vi "Control - Intake Air Desired MAF.vi"(8 "Control Inputs":T1={"Engine Speed [RPM]"=0.0, "Engine Status"=enum."STALLED", "Load Control \nMode"=enum."High-Idle Governor", "dt(s)"=0.0, "Number of Cylinders"=0, "Engine Displacement [cc]"=0.0, "StoichAFR"=0.0, "Q.LHV Fuel [kJ/kg]"=0.0, "BattV PSU [V]"=0.0, "12V PSU [V]"=0.0, "5V PSU [V]"=0.0, "Pedal Position [%]"=0.0, "Oil Pressure [kPa]"=0.0, "Oil Temp [C]"=0.0, "Oil Level [%]"=0.0, "Engine Coolant Temp (ECT) [C]"=0.0, "Engine Coolant Pressure [kPa]"=0.0, "Rail Pressure [bar]"=0.0, "Fuel Pressure [kPa]"=0.0, "Fuel Temp [C]"=0.0, "Vacuum Pressure [kPa]"=0.0, "Throttle Position [%]"=0.0, "Cam1 Advance [CAD]"=0.0, "Cam2 Advance [CAD]"=0.0, "CA50 Control Output [CAD]"=[], "CA50 Control Output Valid"=[], "Intake Air Temp (IAT) [C]"=0.0, "Barometric Air Pressure [kPa]"=0.0, "Intake Air Rel. Humidity [%]"=0.0, "Mass Air Flow (MAF) [kg/hr]"=0.0, "Turbo Inlet Air Pressure [kPa]"=0.0, "Turbo Inlet Air Temp [C]"=0.0, "Turbo Outlet Air Pressure [kPa]"=0.0, "Turbo Outlet Air Temp [C]"=0.0, "CAC Outlet Pressure [kPa]"=0.0, "CAC Outlet Temp [C]"=0.0, "Intake Manifold Pressure (MAP) [kPa]"=0.0, "Intake Manifold Temp (MAT) [C]"=0.0, "Exhaust Manifold Pressure [kPa]"=0.0, "Exhaust Manifold Temp [C]"=0.0, "HighP EGR Cooler Outlet Pressure [kPa]"=0.0, "HighP EGR Cooler Outlet Temp [C]"=0.0, "HighP EGR Differential Pressure [kPa]"=0.0, "HighP EGR Valve Position [%]"=0.0, "Turbo Outlet Exhaust Pressure [kPa]"=0.0, "Turbo Outlet Exhaust Temp [C]"=0.0, "VGT Position 1 [%]"=0.0, "VGT Position 2 [%]"=0.0, "Turbo Speed 1 [RPM]"=0.0, "Turbo Speed 2 [RPM]"=0.0, "LowP EGR Differential Pressure [kPa]"=0.0, "LowP EGR Valve Position [%]"=0.0, "UEGO1Lambda"=0.0, "UEGO1_Hot"=FALSE, "UEGO2Lambda"=0.0, "UEGO2_Hot"=FALSE} {"CA50 Control Output [CAD]" format="%.2f"; "VGT Position 1 [%]" format="%.2f"; "Turbo Speed 2 [RPM]" format="%.2f"; "LowP EGR Valve Position [%]" format="%.2f"; "Turbo Inlet Air Temp [C]" format="%#_6f"; "Turbo Outlet Air Temp [C]" format="%#_6f"; "UEGO2Lambda" format="%.2f"; "Turbo Speed 1 [RPM]" format="%.2f"; "UEGO1Lambda" format="%.2f"}, 9 "Volumetric Efficiency [%]":sgl, 11 "MEP Desired [bar]":sgl) -> (0 "Intake MAP Desired [kPa]":sgl, 1 "Air Mass Desired [mg/cyc]":sgl)   [LabVIEW 2015, in "ECS-RT.lvlib"]
uses:
  ECS-RT.lvlib
  Typedefs/Control Inputs/Control Inputs.ctl
  Typedefs/EPT/Engine Status.ctl
  Typedefs/MISC/Load Control Mode.ctl
  ECS-Shared.lvlib
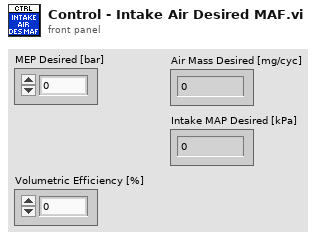
[diagram p1: front panel]
types:
  T1 = typedef "ECS-Shared.lvlib/Control Inputs.ctl" = cluster{"Engine Speed [RPM]":sgl, "Engine Status":T2, "Load Control \nMode":T3, "dt(s)":sgl, "Number of Cylinders":u8, "Engine Displacement [cc]":sgl, "StoichAFR":sgl, "Q.LHV Fuel [kJ/kg]":sgl, "BattV PSU [V]":sgl, "12V PSU [V]":sgl, "5V PSU [V]":sgl, "Pedal Position [%]":sgl, "Oil Pressure [kPa]":sgl, "Oil Temp [C]":sgl, "Oil Level [%]":sgl, "Engine Coolant Temp (ECT) [C]":sgl, "Engine Coolant Pressure [kPa]":sgl, "Rail Pressure [bar]":sgl, "Fuel Pressure [kPa]":sgl, "Fuel Temp [C]":sgl, "Vacuum Pressure [kPa]":sgl, "Throttle Position [%]":sgl, "Cam1 Advance [CAD]":sgl, "Cam2 Advance [CAD]":sgl, "CA50 Control Output [CAD]":sgl[], "CA50 Control Output Valid":bool[], "Intake Air Temp (IAT) [C]":sgl, "Barometric Air Pressure [kPa]":sgl, "Intake Air Rel. Humidity [%]":sgl, "Mass Air Flow (MAF) [kg/hr]":sgl, "Turbo Inlet Air Pressure [kPa]":sgl, "Turbo Inlet Air Temp [C]":sgl, "Turbo Outlet Air Pressure [kPa]":sgl, "Turbo Outlet Air Temp [C]":sgl, "CAC Outlet Pressure [kPa]":sgl, "CAC Outlet Temp [C]":sgl, "Intake Manifold Pressure (MAP) [kPa]":sgl, "Intake Manifold Temp (MAT) [C]":sgl, "Exhaust Manifold Pressure [kPa]":sgl, "Exhaust Manifold Temp [C]":sgl, "HighP EGR Cooler Outlet Pressure [kPa]":sgl, "HighP EGR Cooler Outlet Temp [C]":sgl, "HighP EGR Differential Pressure [kPa]":sgl, "HighP EGR Valve Position [%]":sgl, "Turbo Outlet Exhaust Pressure [kPa]":sgl, "Turbo Outlet Exhaust Temp [C]":sgl, "VGT Position 1 [%]":sgl, "VGT Position 2 [%]":sgl, "Turbo Speed 1 [RPM]":sgl, "Turbo Speed 2 [RPM]":sgl, "LowP EGR Differential Pressure [kPa]":sgl, "LowP EGR Valve Position [%]":sgl, "UEGO1Lambda":sgl, "UEGO1_Hot":bool, "UEGO2Lambda":sgl, "UEGO2_Hot":bool}
  T2 = typedef "ECS-Shared.lvlib/Engine Status.ctl" = enum16{"STALLED", "CRANKING", "RUNNING", "ACCEL", "DECEL", "SAFE", "OFF"}
  T3 = typedef "ECS-Shared.lvlib/Load Control Mode.ctl" = enum16{"No Governor", "Low-Idle Governor", "High-Idle Governor"}
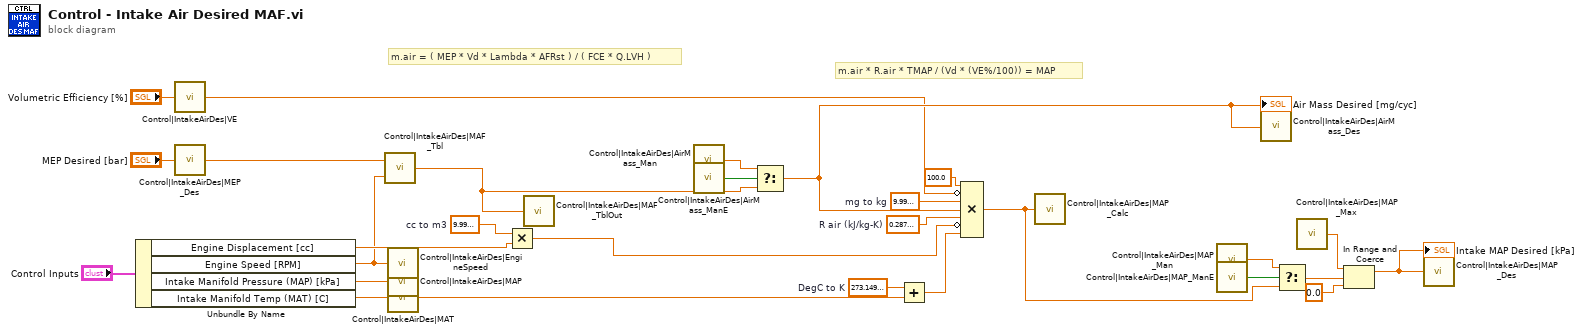
[diagram p0: block diagram]
diagram:
  w12 = sgl 1e-06  # mg to kg
  w8 = sgl 273.15  # DegC to K
  w10 = sgl 0.287  # R air (kJ/kg-K)
  w5 = sgl 1e-06  # cc to m3
  # "m.air * R.air * TMAP / (Vd * (VE%/100)) = MAP"
  # "m.air = ( MEP * Vd * Lambda * AFRst ) / ( FCE * Q.LVH )"
  n1 = Unbundle By Name("Control Inputs") -> ("Engine Displacement [cc]"=w14:sgl, "Engine Speed [RPM]"=w3:sgl, "Intake Manifold Pressure (MAP) [kPa]"=w17:sgl, "Intake Manifold Temp (MAT) [C]"=w15:sgl)
  n2 = call "Control|IntakeAirDes|VE"("Value"="Volumetric Efficiency [%]") -> ()
  n3 = call "Control|IntakeAirDes|MEP_Des"("Value"="MEP Desired [bar]") -> ()
  n4 = call "Control|IntakeAirDes|MAF_Tbl"("Y Index"=w3, "X Index"="MEP Desired [bar]") -> ("Z"=w1:sgl)
  n5 = call "Control|IntakeAirDes|EngineSpeed"("Value"=w3) -> ()
  n6 = call "Control|IntakeAirDes|MAP"("Value"=w17) -> ()
  n7 = call "Control|IntakeAirDes|MAT"("Value"=w15) -> ()
  n8 = Multiply(x=w5, y=w14) -> (x*y=w9:sgl)
  n9 = call "Control|IntakeAirDes|MAF_TblOut"("Value"=w1) -> ()
  n10 = call "Control|IntakeAirDes|AirMass_Man"() -> ("Value"=w6:sgl)
  n11 = call "Control|IntakeAirDes|AirMass_ManE"() -> ("Value"=w7:bool)
  n12 = Select(t=w6, s=w7, f=w1) -> (s? t:f=w19:sgl)
  "Air Mass Desired [mg/cyc]" <- w19
  n13 = Add(x=w8, y=w15) -> (x+y=w11:sgl)
  n14 = Compound Arithmetic op=MULTIPLY(sgl 100.0 ("value"), invert "Volumetric Efficiency [%]", w12, w19, w10, invert w9, w11) -> (w18:sgl)
  n15 = call "Control|IntakeAirDes|MAP_Calc"("Value"=w18) -> ()
  n16 = call "Control|IntakeAirDes|MAP_Man"() -> ("Value"=w21:sgl)
  n17 = call "Control|IntakeAirDes|MAP_ManE"() -> ("Value"=w22:bool)
  n18 = call "Control|IntakeAirDes|AirMass_Des"("Value"=w19) -> ()
  n19 = Select(t=w21, s=w22, f=w18) -> (s? t:f=w20:sgl)
  n20 = call "Control|IntakeAirDes|MAP_Max"() -> ("Value"=w24:sgl)
  n21 = In Range and Coerce(upper limit=w24, x=w20, lower limit=sgl 0.0) -> (coerced(x)=w23:sgl)  [unwired: 1 out]
  "Intake MAP Desired [kPa]" <- w23
  n22 = call "Control|IntakeAirDes|MAP_Des"("Value"=w23) -> ()
